vi "MCB2400 Button PrjAttrValidator.vi"(5 "Ctl Refnum":refnum<vi>, 9 "IO channel number":u32(ring) items=["0", "1", "2", "3", "4", "5", "6", "7"], 11 "Attributes":T1 {"Programmable Pin Connections" items=["Button4 and LED4 use the same pin P2.10. You cannot use Button4 and LED4 in the same project.", "Button0-3 and LED0-3 use pins P0.27 and P0.28.  You cannot use Button0-3, LED0-3, P0.27, or P0.28 in the same project."]}) -> (3 "Valid?":bool)   [LabVIEW 2011]
uses:
  <vilib>/Embedded/ARM/MCB2400/MCB2400_Button_PrjAttr.ctl
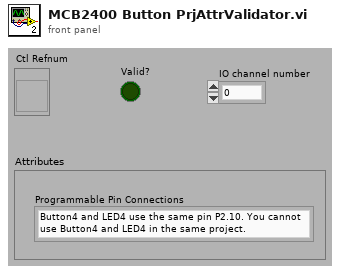
[diagram p1: front panel]
types:
  T1 = typedef "MCB2400_Button_PrjAttr.ctl" = cluster{"Programmable Pin Connections":u16}
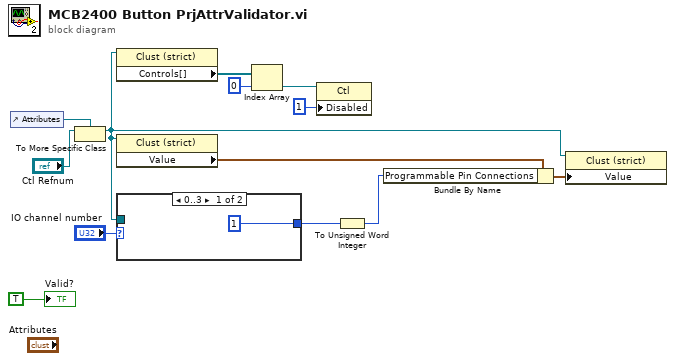
[diagram p0: block diagram]
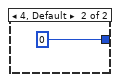
[diagram p2: hidden frame]
diagram:
  n1 = control-ref of="Attributes"() -> (w2:refnum<vi>)
  n2 = To More Specific Class(target class=w2, reference="Ctl Refnum") -> (specific class reference=w5:refnum<vi>)  [unwired: 1 in, 1 out]
  n3 = property class="Clust (strict)"(reference=w5) -> ("Controls[]"=w10:refnum<vi>[])  [unwired: 1 in, 2 out]
  n4 = property class="Clust (strict)"(reference=w5) -> ("Value"=w12:cluster{"Programmable Pin Connections":u16})  [unwired: 1 in, 2 out]
  n5 = case shown="0..3" "IO channel number" {
    tunnel: [u32 1 u32 0] -> w6
    tunnel: w5 -> [_ _]
    frame 0..3 {
    }
    frame 4, Default {
    }
  }
  n6 = Index Array(array=w10, index=0) -> (element=w8:refnum<vi>)
  n7 = property class="Ctl"(reference=w8, "Disabled"=u8 1) -> ()  [unwired: 1 in, 2 out]
  n8 = To Unsigned Word Integer(number=w6) -> (unsigned 16bit integer=w1:u16)
  n9 = Bundle By Name(cluster=w12, "Programmable Pin Connections"=w1) -> (w11:cluster{"Programmable Pin Connections":u16})
  n10 = property class="Clust (strict)"(reference=w5, "Value"=w11) -> ()  [unwired: 1 in, 2 out]
  "Valid?" <- TRUE ("Valid?")
